vi "UpdateCVT[Acquire].vi"(8 "error in (no error)":errorcluster, 11 "GenericCamera in":refnum<class "GenericCamera.lvclass">) -> (0 "error out":errorcluster, 3 "GenericCamera out":refnum<class "GenericCamera.lvclass">)   [LabVIEW 2013, in "GenericCamera.lvclass"]
uses:
  GenericCamera.lvclass
  CompressAndUpdate(Poly)/CompressAndUpdate(Numeric).vi
  CompressAndUpdate(Poly)/CompressAndUpdate(IMAQ Image).vi
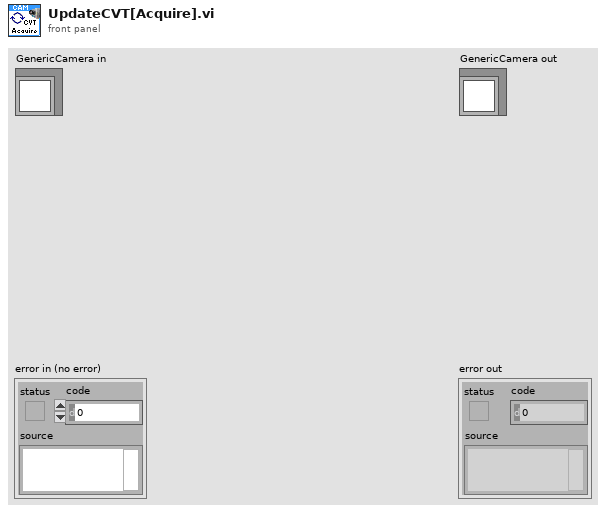
[diagram p1: front panel]
types:
  T1 = typedef "IMAQ Image.ctl" = refnum<image>
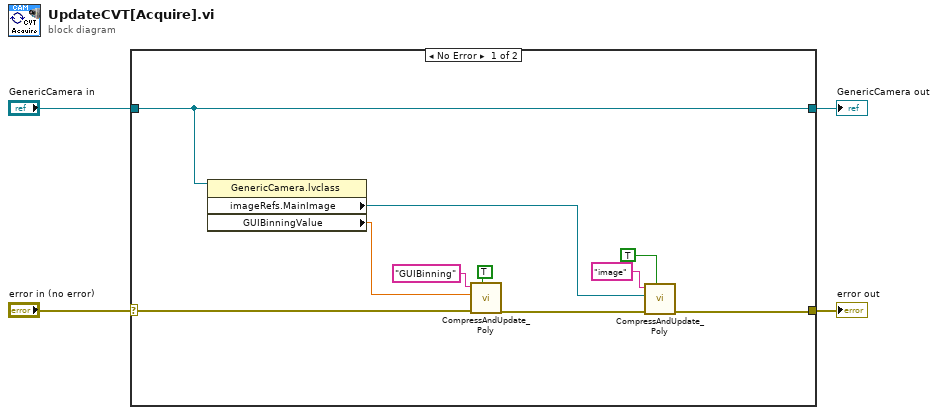
[diagram p0: block diagram]
diagram:
  n1 = case shown="No Error" "error in (no error)" {
    selector: "error in (no error)" -> [w7 w16]
    tunnel: [w5 w16] -> w3
    tunnel: [w8 w15] -> w1
    tunnel: "GenericCamera in" -> [w8 w15]
    frame No Error {
      n2 = property class="GenericCamera.lvclass"(reference=w8) -> ("imageRefs.MainImage"=w13:T1, "GUIBinningValue"=w6:dbl)  [unwired: 1 in, 2 out]
      n3 = call-poly "CompressAndUpdate_Poly.vi"("force CVT update (false)"=TRUE, "error in"=w7, "Numeric"=w6, "command or variable name"="GUIBinning") -> ("error out"=w10:errorcluster)  [unwired: 7 in]
      n4 = call-poly "CompressAndUpdate_Poly.vi"("force CVT update (false)"=TRUE, "error in"=w10, "IMAQ Image"=w13, "command or variable name"="image") -> ("error out"=w5:errorcluster)  [unwired: 7 in]
    }
    frame Error {
    }
  }
  "error out" <- w3
  "GenericCamera out" <- w1
